vi "GenerateCLZSeriesMap.vi"(7 "key set":set{cluster{"clz.key":i32, "marvel.key":i32}}(c389), 8 "error in (no error)":errorcluster, 11 "map in":T1(c390)) -> (0 "error out":errorcluster, 3 "series map":T1(c390))   [LabVIEW 2024]
uses:
  <vilib>/Utility/file.llb/Read Delimited Spreadsheet (string).vi
panel:
  out "all rows":string[][](array[string])
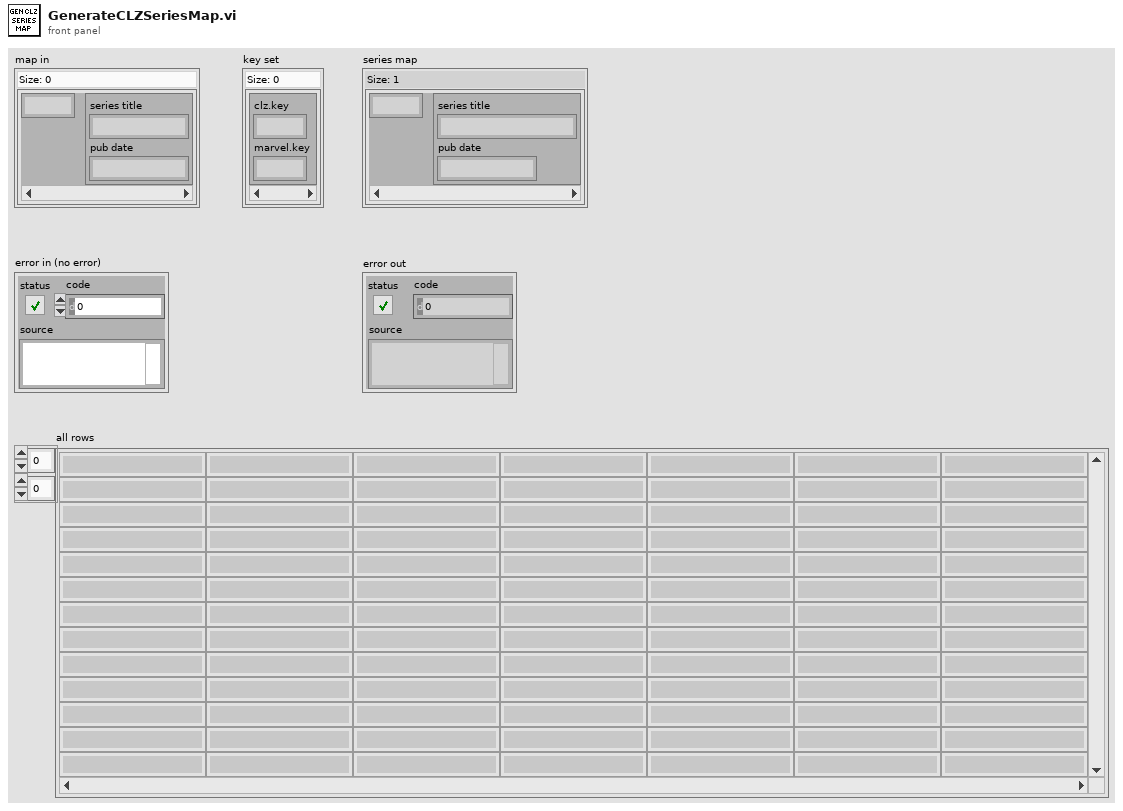
[diagram p1: front panel]
types:
  T1 = map{i32, cluster{"series title":string, "pub date":string}}
  T2 = cluster{"series title":string, "pub date":string}
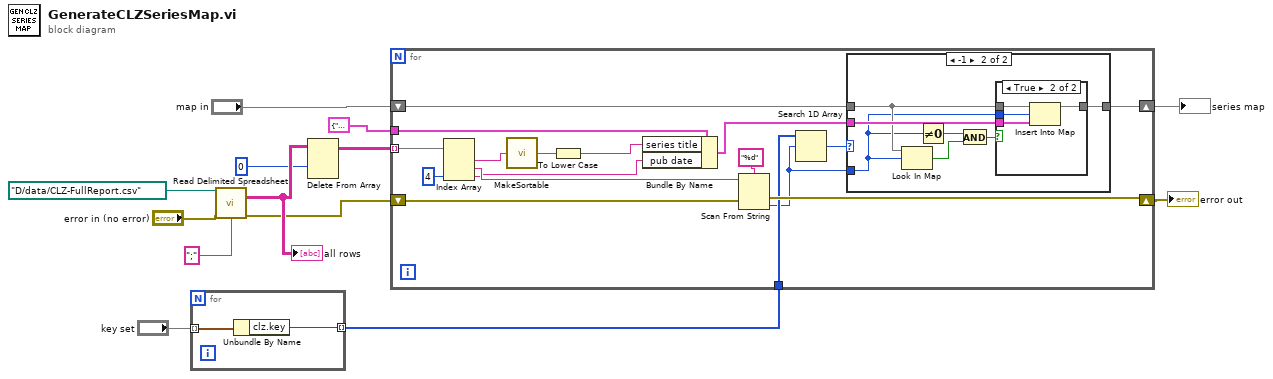
[diagram p0: block diagram]
diagram:
  n1 = for {
    tunnel: "key set" -> [w15] mode=indexing
    tunnel: [w14] -> w1 mode=indexing
    n2 = Unbundle By Name(w15) -> ("clz.key"=w14:i32)
  }
  n3 = call-poly <vilib>:"Read Delimited Spreadsheet.vi"("file path (dialog if empty)"=path "D:/data/CLZ-FullReport.csv", "error in (no error)"="error in (no error)", "delimiter (\\t)"=";" ("delimiter (\\t)")) -> ("all rows"=w11:string[][], "error out"=w8:errorcluster)  [unwired: 7 in, 4 out]
  "all rows" <- w11
  n4 = Delete From Array(array=w11, index (row)=0) -> (array with subset deleted=w9:string[][])  [unwired: 2 in, 1 out]
  n5 = for {
    tunnel: w9 -> [w32] mode=indexing
    shift-right: [w29] -> w7
    shift-left: w8 -> [w30]
    shift-right: [w27] -> w6
    shift-left: "map in" -> [w22]
    tunnel: T2 {"series title"="", "pub date"=""} -> [w25]
    tunnel: w1 -> [w18]
    n6 = Index Array(array=w32, index #3=4 ("index")) -> (element #1=w21:string, element #2=w28:string, element #3=w24:string)  [unwired: 2 in]
    n7 = call "MakeSortable.vi"("string in"=w21) -> ("string out"=w20:string)
    n8 = To Lower Case(string=w20) -> (all lower case string=w19:string)
    n9 = Bundle By Name(cluster=w25, "series title"=w19, "pub date"=w24) -> (w23:T2)
    n10 = Scan From String(format string="%d", input string=w28, error in=w30) -> (error out=w29:errorcluster, output 1=w17:i32)  [unwired: 2 in, 2 out]
    n11 = Search 1D Array(1D array=w18, element=w17) -> (index of element=w16:i32)  [unwired: 1 in]
    n12 = case shown="-1" w16 {
      tunnel: [w33 w40] -> w27
      tunnel: w23 -> [_ w39]
      tunnel: w22 -> [w33 w38]
      tunnel: w17 -> [_ w34]
      frame Default {
      }
      frame -1 {
        n13 = Look In Map(map=w38, key=w34) -> (key not found?=w36:bool)  [unwired: 1 in, 1 out]
        n14 = Not Equal To 0?(x=w34) -> (x != 0?=w35:bool)
        n15 = And(x=w35, y=w36) -> (x .and. y?=w37:bool)
        n16 = case shown="True" w37 {
          tunnel: [w41 w45] -> w40
          tunnel: w39 -> [_ w44]
          tunnel: w38 -> [w41 w43]
          tunnel: w34 -> [_ w42]
          frame False {
          }
          frame True {
            n17 = Insert Into Map(map in=w43, key=w42, value=w44) -> (map out=w45:T1)  [unwired: 2 out]
          }
        }
      }
    }
  }
  "error out" <- w7
  "series map" <- w6
